vi "High-Level Write to Text File - N-Channel.vi"() -> ()   [LabVIEW 2019]
uses:
  <vilib>/DAQmx/read.llb/DAQmx Read (Analog 2D DBL NChan NSamp).vi
  <vilib>/DAQmx/create/channels.llb/DAQmx Create Channel (AI-Voltage-Basic).vi
  <vilib>/DAQmx/configure/timing.llb/DAQmx Timing (Sample Clock).vi
  <vilib>/DAQmx/miscellaneous.llb/DAQmx Fill In Error Info.vi
  <resource>/objmgr/daqmx.rc
panel:
  in  "minimum value":dbl=-5.0
  in  "maximum value":dbl=5.0
  out "Waveform Graph":dbl[][](graph)
  in  "Number of Samples":i32=100
  in  "Desired Sample Rate (Hz)":dbl=1000.0
  in  "Physical Channel":tag="PCI-6221/ai0:3"
  out "Actual Sample Rate (Hz)":dbl
  # "Measurement Range"
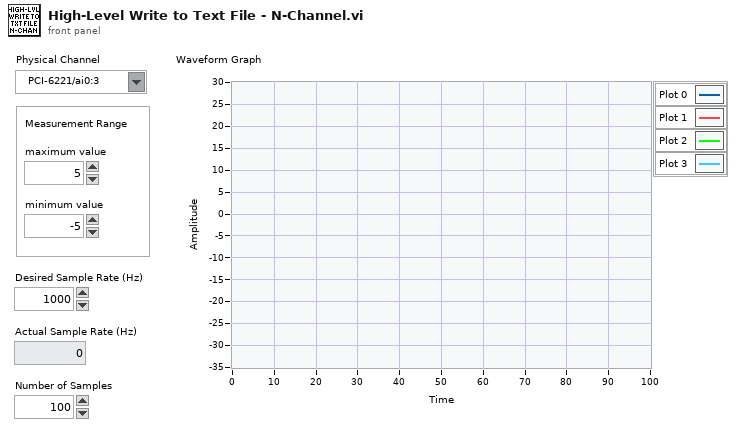
[diagram p1: front panel]
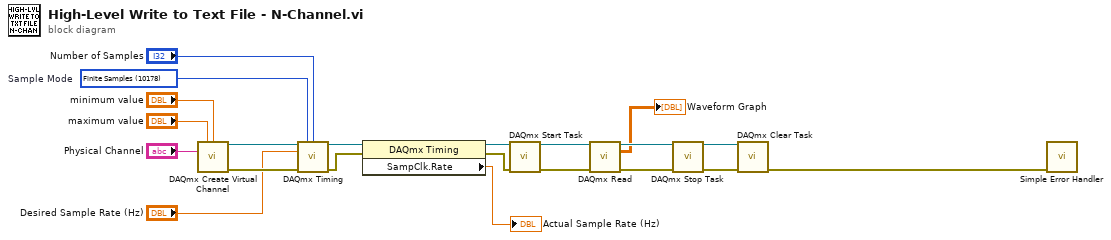
[diagram p0: block diagram]
diagram:
  w13 = 10178 items=["Finite Samples"=10178, "Continuous Samples"=10123, "Hardware Timed Single Point"=12522]  # Sample Mode
  n1 = call-poly <vilib>:"DAQmx Create Virtual Channel.vi"("maximum value"="maximum value", "minimum value"="minimum value", "physical channels"="Physical Channel") -> ("task out"=w21:refnum<k21>, "error out"=w20:errorcluster)  [unwired: 11 in]
  n2 = call-poly <vilib>:"DAQmx Timing.vi"("task/channels in"=w21, "sample mode"=w13, "samples per channel"="Number of Samples", "rate"="Desired Sample Rate (Hz)", "error in"=w20) -> ("task out"=w19:refnum<k21>, "error out"=w18:errorcluster)  [unwired: 9 in]
  n3 = property class="DAQmx Timing"(reference=w19, error in=w18) -> (reference out=w17:refnum<k21>, error out=w16:errorcluster, "SampClk.Rate"=→"Actual Sample Rate (Hz)":dbl)
  n4 = call <vilib>:"DAQmx Start Task.vi"("task/channels in"=w17, "error in"=w16) -> ("task out"=w15:refnum<k21>, "error out"=w14:errorcluster)  [unwired: 12 in]
  n5 = call-poly <vilib>:"DAQmx Read.vi"("task/channels in"=w15, "error in"=w14) -> ("task out"=w12:refnum<k21>, "data"=→"Waveform Graph":dbl[][], "error out"=w11:errorcluster)  [unwired: 11 in]
  n6 = call <vilib>:"DAQmx Stop Task.vi"("task/channels in"=w12, "error in"=w11) -> ("task out"=w10:refnum<k21>, "error out"=w9:errorcluster)  [unwired: 12 in]
  n7 = call <vilib>:"DAQmx Clear Task.vi"("task in"=w10, "error in"=w9) -> ("error out"=w1:errorcluster)  [unwired: 13 in]
  n8 = call <vilib>:"Simple Error Handler.vi"("error in (no error)"=w1) -> ()  [unwired: 4 in, 5 out]
